vi "PSLDAQ_Open.vi"(1 "DeviceID":string) -> (0 "Handle Out":T1)   [LabVIEW 2010]
doc: "1. 설명\n a. 장치와의 통신 연결 기능을 활성화하며, PSLDAQ_Dll을 동작시키기 위한 초기화 및 메모리 할당\n\n2. 기능\n a. PSLDAQ_Dll.dll의 기능과 관련된 메모리 할당/Thread 생성 등의 초기화 \n b. PSL-DAQ 장치와 통신 연결 기능 활성화\n c. 다른 함수에서 사용할 장치 핸들 생성 \n ※ PSL-DAQ LabVIEW Library를 사용하기 위한 필수 함수 \n\n3. 터미널\n a. 터미널 입력\n ○ DeviceID :\n - 연결할 PSL DAQ 장치의 ID 이며,PSLDAQ_GetDeviceID VI를 통해 얻을 수 있다.\n ㆍPDAQ-xxxxxxx(PDAQ-7자리숫자) \n - PSL-DAQ 장치가 PC에 1대 연결된 경우 \n ㆍDeviceID를 빈 문자열로 입력 - 연결된 PSL-DAQ 장치의 DeviceID를 자동으로 읽어 \n 통신 연결 활성화\n ㆍDeviceID에 장치 ID를 입력 - 입력된 DeviceID와 일치하는 PSL-DAQ 장치만 \n 통신 연결 활성화 \n - PSL-DAQ 장치가 PC에 여러대 연결된 경우 \n ㆍDeviceID를 빈 문자열로 입력 - “Device Selection Dialog\" 창에 여러 DeviceID가\n 표시되며, 연결할 장치의 ID를 선택하여 통신 연결 활성화\n ㆍDeviceID에 장치 ID를 입력 - 입력된 DeviceID와 일치하는 PSL DAQ 장치만 통신 연결 활성화.\n “Device Selection Dialog\"는 나타나지 않음\n\n b. 터미널 출력\n ○ Handle Out\n - 장치 핸들, PSLDAQ_Open VI를 제외한 모든 VI에 사용되어짐 \n - PSLDAQ_Open VI를 사용해 연결된 PSL DAQ 장치에서 데이터 획득 등에 사용됨\n\n4. 주의\n a. PSLDAQ_Open VI를 사용한 경우 반드시 PSLDAQ_Close VI를 사용해야 함. \n b. DeviceID를 부정확하게 입력하면 장치가 열리지 않음. \n c. 여러 대(n 대)의 PSL DAQ 장치를 LabVIEW에서 사용할 경우에는 PSLDAQ_Open 함수를 \n n번 호출하여 n개의 장치 핸들을 생성해야 한다. 또한 n개의 PSLDAQ_Close도 호출해야 함.\n d. 여러 대의 PSL-DAQ 장치가 PC에 연결된 경우에 각각의 PSLDAQ_Open 함수에 DeviceID를\n 기록해서 사용하기를 권장함."
uses:
  PSLDAQ_Dll.dll
panel:
  # "PSLDAQ_Open\n\n1. 설명\n  a. 장치와의 통신 연결 기능을 활성화하며, PSLDAQ_Dll을 동작시키기 위한 초기화 및 메모리 할당\n\n2. 기능\n  a. PSLDAQ_Dll.dll의 기능과 관련된 메모리 할당/Thread 생성 등의 초기화 \n  b. PSL-DAQ 장치와 통신 연결 기능 활성화\n  c. 다른 함수에서 사용할 장치 핸들 생성        \n  ※ PSL-DAQ LabVIEW Library를 사용하기 위한 필수 함수 \n\n3. 터미널\n  a. 터미널 입력\n     ○ DeviceID :\n        - 연결할 PSL DAQ 장치의 ID 이며,PSLDAQ_GetDeviceID VI를 통해 얻을 수 있다.\n        ㆍPDAQ-xxxxxxx(PDAQ-7자리숫자) \n        - PSL-DAQ 장치가 PC에 1대 연결된 경우 \n        ㆍDeviceID를 빈 문자열로 입력 - 연결된 PSL-DAQ 장치의 DeviceID를 자동으로 읽어 \n           통신 연결 활성화\n        ㆍDeviceID에 장치 ID를 입력 - 입력된 DeviceID와 일치하는 PSL-DAQ 장치만  \n           통신 연결 활성화     \n        - PSL-DAQ 장치가 PC에 여러대 연결된 경우 \n        ㆍDeviceID를 빈 문자열로 입력 - “Device Selection Dialog\" 창에 여러 DeviceID가\n           표시되며, 연결할 장치의 ID를 선택하여 통신 연결 활성화\n        ㆍDeviceID에 장치 ID를 입력 - 입력된 DeviceID와 일치하는 PSL DAQ 장치만  통신 연결 활성화.\n           “Device Selection Dialog\"는 나타나지 않음\n\n  b. 터미널 출력\n     ○ Handle Out\n        - 장치 핸들, PSLDAQ_Open VI를 제외한 모든 VI에 사용되어짐 \n        - PSLDAQ_Open VI를 사용해 연결된 PSL DAQ 장치에서 데이터 획득 등에 사용됨\n\n4. 주의\n  a. PSLDAQ_Open VI를 사용한 경우 반드시 PSLDAQ_Close VI를 사용해야 함.  \n  b. DeviceID를 부정확하게 입력하면 장치가 열리지 않음. \n  c. 여러 대(n 대)의 PSL DAQ 장치를 LabVIEW에서 사용할 경우에는 PSLDAQ_Open 함수를 \n      n번 호출하여  n개의 장치 핸들을 생성해야 한다. 또한 n개의 PSLDAQ_Close도 호출해야 함.\n  d. 여러 대의 PSL-DAQ 장치가 PC에 연결된 경우에 각각의 PSLDAQ_Open 함수에 DeviceID를\n      기록해서 사용하기를 권장함."
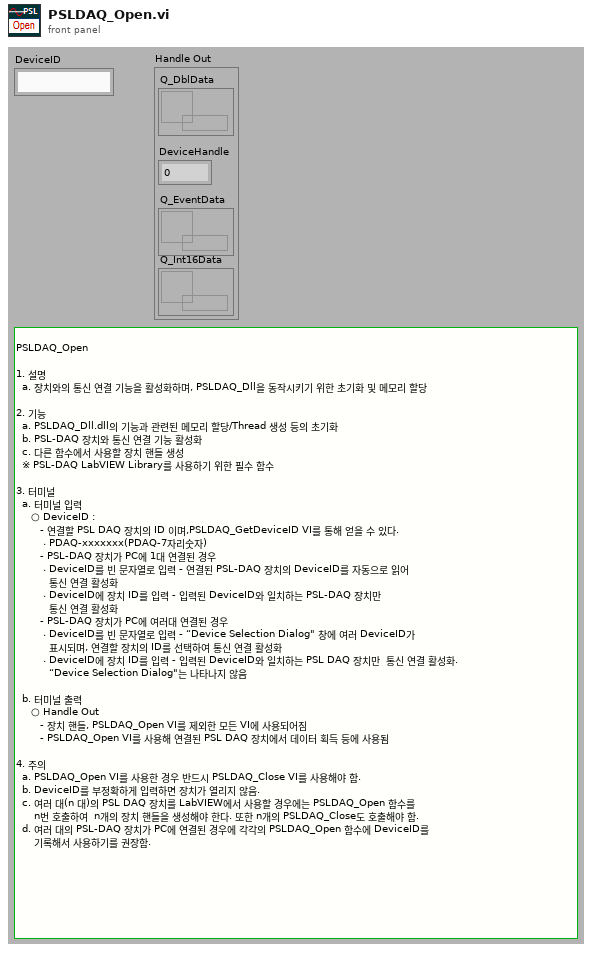
[diagram p1: front panel]
types:
  T1 = cluster{"Q_DblData":refnum<queue>, "DeviceHandle":u32, "Q_EventData":refnum<queue>, "Q_Int16Data":refnum<queue>}
  T2 = cluster{"queue out":refnum<queue>, "DeviceHandle":u32, "queue out":refnum<queue>, "queue out":refnum<queue>}
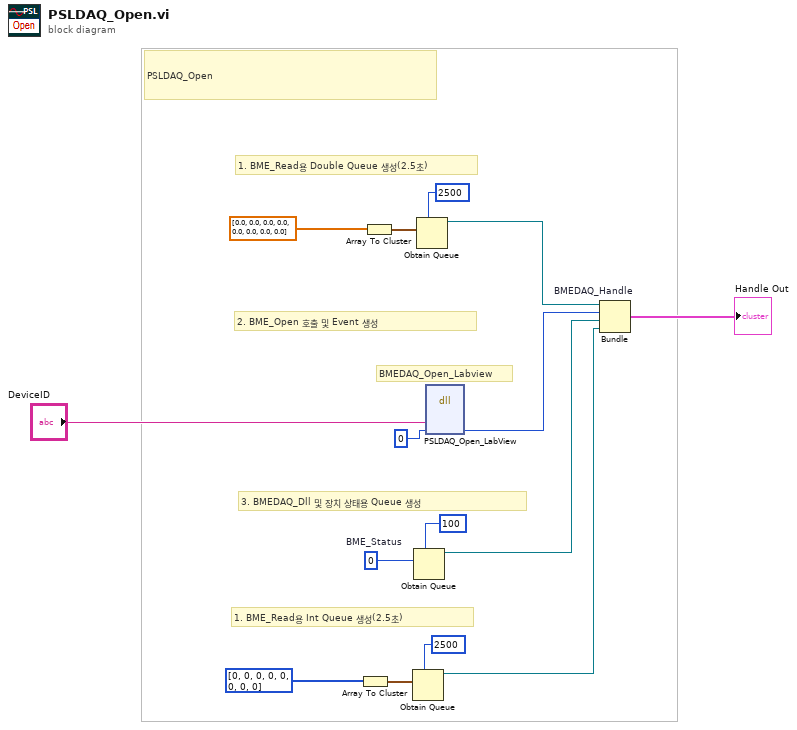
[diagram p0: block diagram]
diagram:
  w13 = u32 0  # BME_Status
  # "1. BME_Read용 Int Queue 생성(2.5초)"
  # "BMEDAQ_Open_Labview"
  # "3. BMEDAQ_Dll 및 장치 상태용 Queue 생성"
  # "PSLDAQ_Open"
  # "2. BME_Open 호출 및 Event 생성"
  # "1. BME_Read용 Double Queue 생성(2.5초)"
  n1 = Array To Cluster(array=i16[] [0, 0, 0, 0, 0, 0, 0, 0]) -> (cluster=w5:cluster{"[0]":i16, "[1]":i16})
  n2 = Array To Cluster(array=dbl[] [0.0, 0.0, 0.0, 0.0, 0.0, 0.0, 0.0, 0.0]) -> (cluster=w9:cluster{"[0]":dbl, "[1]":dbl})
  n3 = Obtain Queue(max queue size (-1, unlimited)=2500, element data type=w5) -> (queue out=w2:refnum<queue>)  [unwired: 3 in, 2 out]
  n4 = Obtain Queue(max queue size (-1, unlimited)=100, element data type=w13) -> (queue out=w12:refnum<queue>)  [unwired: 3 in, 2 out]
  n5 = Obtain Queue(max queue size (-1, unlimited)=2500, element data type=w9) -> (queue out=w10:refnum<queue>)  [unwired: 3 in, 2 out]
  n6 = dll-call lib="D:/PSL-DAQ LabVIEW Library/PSLDAQ_Dll.dll" fn="PSLDAQ_Open_LabView"("DeviceName"="DeviceID", "DeviceHandle"=u32 0) -> ("DeviceHandle"=w14:u32)  [unwired: 7 in, 2 out]
  n7 = Bundle "BMEDAQ_Handle"("queue out"=w10, "DeviceHandle"=w14, "queue out"=w12, "queue out"=w2) -> (→"Handle Out":T2)  [unwired: 1 in]
